vi "labview4.vi"() -> ()   [LabVIEW 2019]
uses:
  <vilib>/addons/eal4LabVIEW/ApiLib/Connection control/ealApiConnect_string.vi
  <vilib>/Utility/inputDevices.llb/joystickAcquire.vi
  <vilib>/Utility/inputDevices.llb/closeJoystick.vi
  <vilib>/addons/eal4LabVIEW/eal4LabVIEW.lvlib
panel:
  out "appended array":bool[](array[boolean])
  out "In Range? (1)":bool
  out "In Range? (2)":bool
  out "In Range? (3)":bool
  in  "condition 6":i32(ring) items=["AXIS_CONDITION_ACTIVE"=0, "AXIS_CONDITION_PARKING"=1, "AXIS_CONDITION_DEACTIVATED"=2, "AXIS_CONDITION_ACTIVE_DECOUPLED"=4, "AXIS_CONDITION_PARKING_DECOUPLED"=5, "AXIS_CONDITION_DEACTIVATED_DECOUPLED"=6, "AXIS_CONDITION_ACTIVE_PARAMETERIZATION"=8, "AXIS_CONDITION_PARKING_PARAMETERIZATION"=9, "AXIS_CONDITION_DEACTIVATED_PARAMETERIZATION"=10, "AXIS_CONDITION_ACTIVE_DECOUPLED_PARAMETERIZATION"=12, "AXIS_CONDITION_PARKING_DECOUPLED_PARAMETERIZATION"=13, "AXIS_CONDITION_DEACTIVATED_DECOUPLED_PARAMETERIZATION"=14]
  in  "slave index 6":i32
  in  "condition 5":i32(ring) items=["AXIS_CONDITION_ACTIVE"=0, "AXIS_CONDITION_PARKING"=1, "AXIS_CONDITION_DEACTIVATED"=2, "AXIS_CONDITION_ACTIVE_DECOUPLED"=4, "AXIS_CONDITION_PARKING_DECOUPLED"=5, "AXIS_CONDITION_DEACTIVATED_DECOUPLED"=6, "AXIS_CONDITION_ACTIVE_PARAMETERIZATION"=8, "AXIS_CONDITION_PARKING_PARAMETERIZATION"=9, "AXIS_CONDITION_DEACTIVATED_PARAMETERIZATION"=10, "AXIS_CONDITION_ACTIVE_DECOUPLED_PARAMETERIZATION"=12, "AXIS_CONDITION_PARKING_DECOUPLED_PARAMETERIZATION"=13, "AXIS_CONDITION_DEACTIVATED_DECOUPLED_PARAMETERIZATION"=14]
  in  "slave index 5":i32
  in  "condition 4":i32(ring) items=["AXIS_CONDITION_ACTIVE"=0, "AXIS_CONDITION_PARKING"=1, "AXIS_CONDITION_DEACTIVATED"=2, "AXIS_CONDITION_ACTIVE_DECOUPLED"=4, "AXIS_CONDITION_PARKING_DECOUPLED"=5, "AXIS_CONDITION_DEACTIVATED_DECOUPLED"=6, "AXIS_CONDITION_ACTIVE_PARAMETERIZATION"=8, "AXIS_CONDITION_PARKING_PARAMETERIZATION"=9, "AXIS_CONDITION_DEACTIVATED_PARAMETERIZATION"=10, "AXIS_CONDITION_ACTIVE_DECOUPLED_PARAMETERIZATION"=12, "AXIS_CONDITION_PARKING_DECOUPLED_PARAMETERIZATION"=13, "AXIS_CONDITION_DEACTIVATED_DECOUPLED_PARAMETERIZATION"=14]
  in  "slave index 4":i32
  out "RPM Motor 1":dbl
  out "RPM Motor 2":dbl
  out "RPM Motor 3":dbl
  in  "stop":bool
  out "return value":dbl[](array[numeric])
  out "Iteration counter":i32
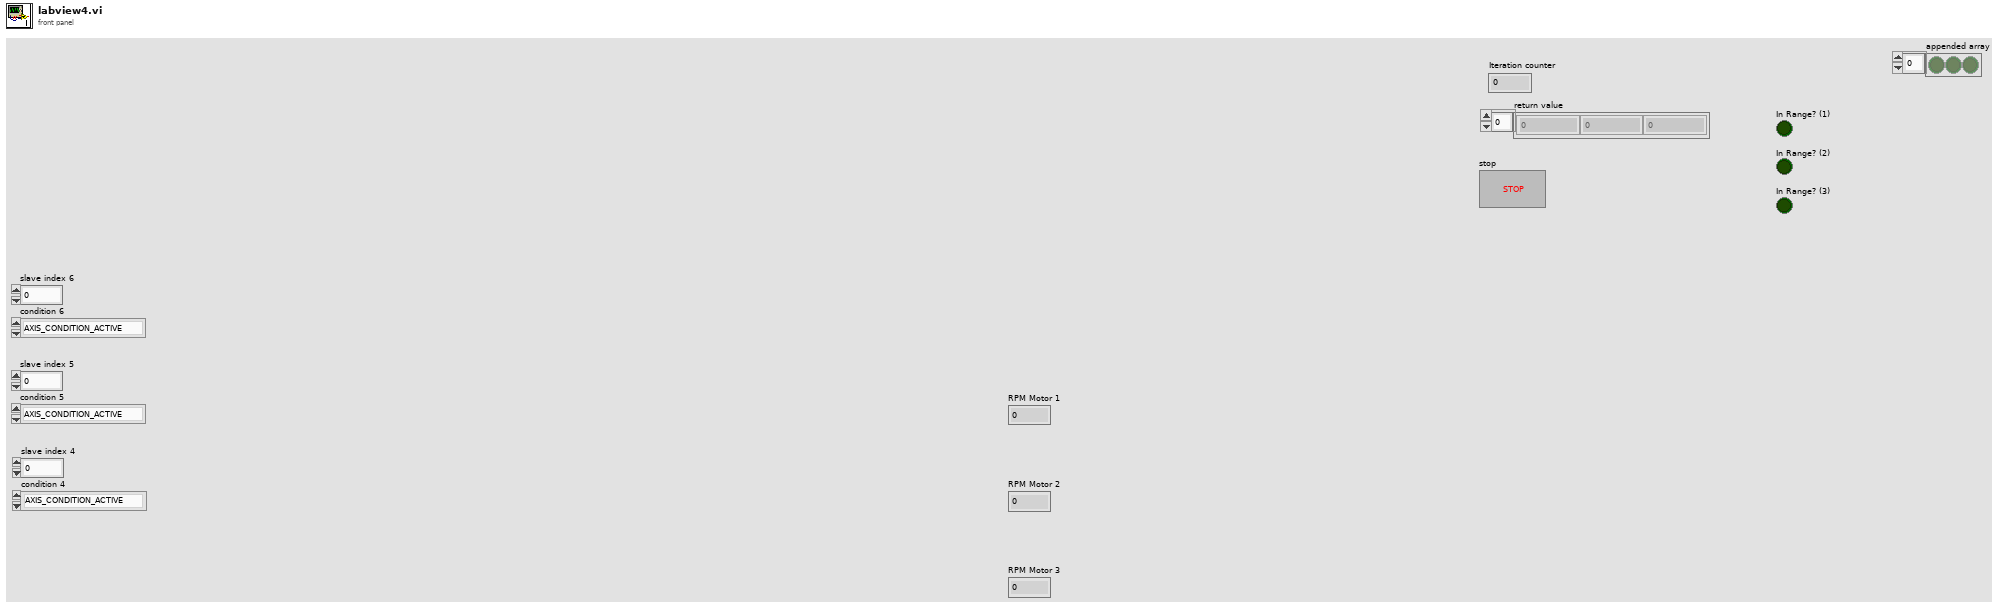
[diagram p1: front panel]
types:
  T1 = cluster{"Velocity":dbl, "Acceleration":dbl, "Deceleration":dbl, "Jerk":dbl}
  T2 = cluster{"X axis":i32, "Y axis":i32, "Z axis":i32, "X axis rotation":i32, "Y axis rotation":i32, "Z axis rotation":i32, "U axis":i32, "V axis":i32}
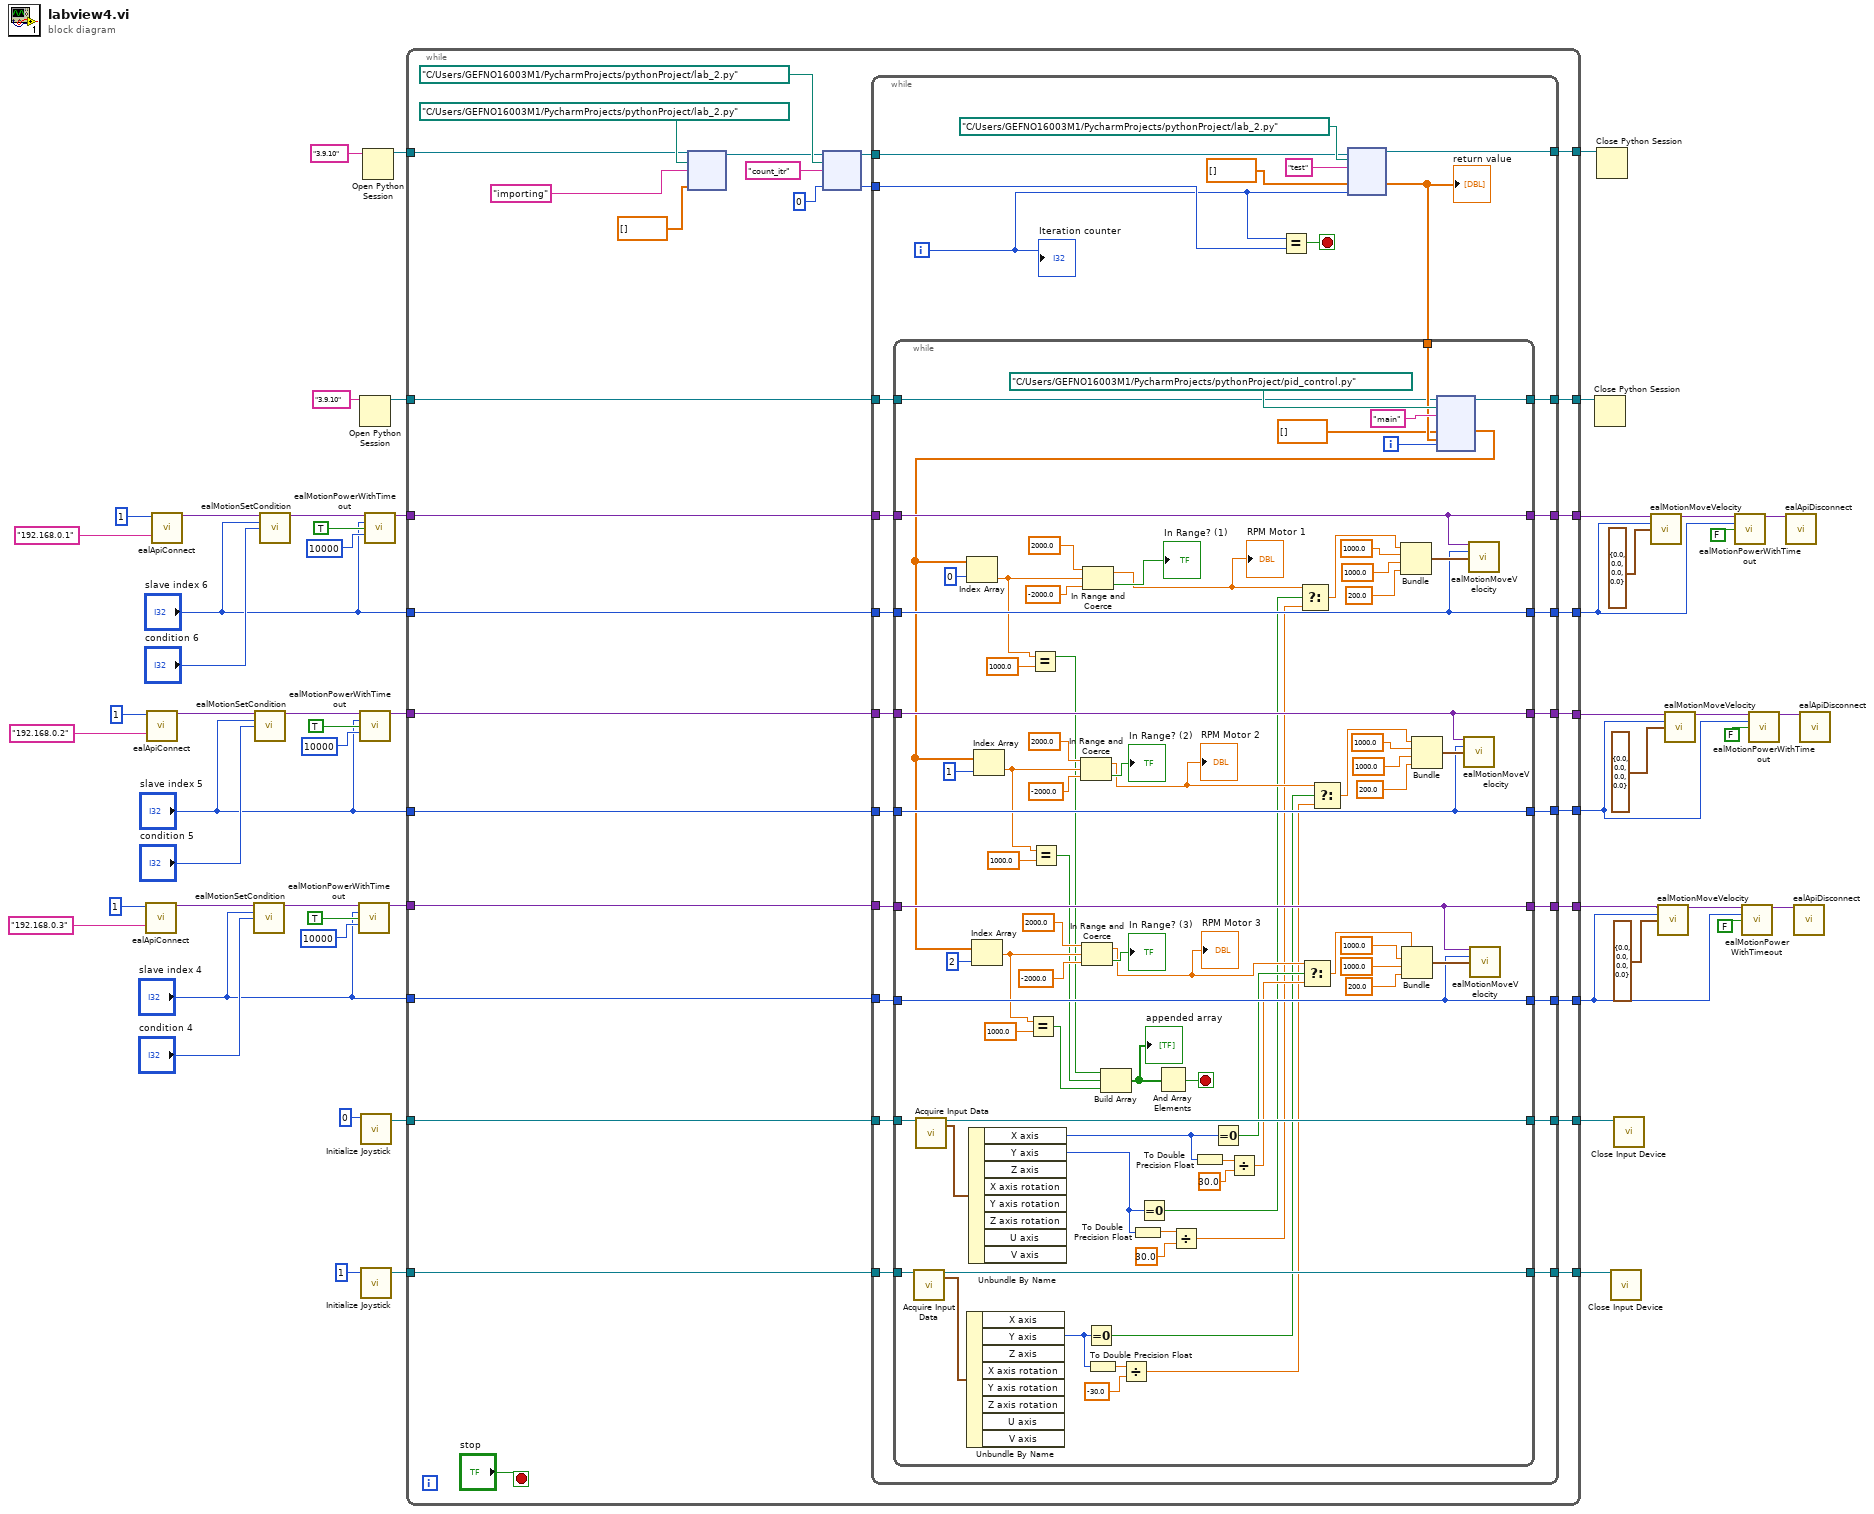
[diagram p0: block diagram]
diagram:
  n1 = call-poly <vilib>:"ealApiConnect.vi"("maximum no of axes"=1, "ip address"="192.168.0.3") -> ("connection out"=w43:variant)  [unwired: 12 in, 1 out]
  n2 = call-poly <vilib>:"ealApiConnect.vi"("maximum no of axes"=1, "ip address"="192.168.0.2") -> ("connection out"=w36:variant)  [unwired: 12 in, 1 out]
  n3 = call-poly <vilib>:"ealApiConnect.vi"("maximum no of axes"=1, "ip address"="192.168.0.1") -> ("connection out"=w29:variant)  [unwired: 12 in, 1 out]
  n4 = call <vilib>:"ealMotionSetCondition.vi"("connection in"=w43, "slave index"="slave index 4", "condition"="condition 4") -> ("connection out"=w42:variant)  [unwired: 11 in, 1 out]
  n5 = call <vilib>:"ealMotionSetCondition.vi"("connection in"=w36, "slave index"="slave index 5", "condition"="condition 5") -> ("connection out"=w35:variant)  [unwired: 11 in, 1 out]
  n6 = call <vilib>:"ealMotionSetCondition.vi"("connection in"=w29, "slave index"="slave index 6", "condition"="condition 6") -> ("connection out"=w28:variant)  [unwired: 11 in, 1 out]
  n7 = call <vilib>:"ealMotionPowerWithTimeout.vi"("connection in"=w42, "slave index"="slave index 4", "value"=TRUE, "timeout"=10000) -> ("connection out"=w22:variant)  [unwired: 10 in, 1 out]
  n8 = Open Python Session(python version="3.9.10" ("Python version")) -> (session out=w10:refnum<k35>)  [unwired: 2 in, 1 out]
  n9 = call <vilib>:"ealMotionPowerWithTimeout.vi"("connection in"=w35, "slave index"="slave index 5", "value"=TRUE, "timeout"=10000) -> ("connection out"=w23:variant)  [unwired: 10 in, 1 out]
  n10 = call <vilib>:"Initialize Joystick.vi"("device index"=0) -> ("device ID"=w4:refnum<k1>)  [unwired: 9 in, 1 out]
  n11 = call <vilib>:"Initialize Joystick.vi"("device index"=1) -> ("device ID"=w3:refnum<k1>)  [unwired: 9 in, 1 out]
  n12 = Open Python Session(python version="3.9.10" ("Python version")) -> (session out=w13:refnum<k35>)  [unwired: 2 in, 1 out]
  n13 = call <vilib>:"ealMotionPowerWithTimeout.vi"("connection in"=w28, "slave index"="slave index 6", "value"=TRUE, "timeout"=10000) -> ("connection out"=w24:variant)  [unwired: 10 in, 1 out]
  n14 = while {
    tunnel: w24 -> [w77]
    tunnel: w23 -> [w76]
    tunnel: w22 -> [w75]
    tunnel: [w74] -> w21
    tunnel: [w73] -> w20
    tunnel: "slave index 6" -> [w72]
    tunnel: "slave index 5" -> [w71]
    tunnel: [w70] -> w17
    tunnel: [w63] -> w16
    tunnel: "slave index 4" -> [w69]
    tunnel: w13 -> [w68]
    tunnel: [w67] -> w12
    tunnel: w10 -> [w66]
    tunnel: [w65] -> w9
    tunnel: [w64] -> w8
    tunnel: [w62] -> w7
    tunnel: w4 -> [w61]
    tunnel: w3 -> [w60]
    tunnel: [w59] -> w2
    tunnel: [w58] -> w1
    stop <- "stop" stop-if-true
    n15 = node(w68, path "C:/Users/GEFNO16003M1/PycharmProjects/pythonProject/lab_2.py" ("module path"), "importing" ("function name"), dbl[] []) -> (w82:refnum<k35>)  [unwired: 2 in, 3 out]
    n16 = node(w82, path "C:/Users/GEFNO16003M1/PycharmProjects/pythonProject/lab_2.py" ("module path"), "count_itr" ("function name"), 0) -> (w81:refnum<k35>, w79:i32)  [unwired: 1 in, 3 out]
    n17 = while {
      tunnel: [w108] -> w67
      tunnel: w81 -> [w111]
      tunnel: w79 -> [w109]
      tunnel: w77 -> [w106]
      tunnel: w76 -> [w95]
      tunnel: w75 -> [w105]
      tunnel: [w97] -> w74
      tunnel: [w98] -> w73
      tunnel: w72 -> [w96]
      tunnel: w71 -> [w94]
      tunnel: [w99] -> w70
      tunnel: w69 -> [w101]
      tunnel: w66 -> [w93]
      tunnel: [w103] -> w65
      tunnel: [w102] -> w64
      tunnel: [w100] -> w63
      tunnel: [w92] -> w62
      tunnel: w61 -> [w91]
      tunnel: w60 -> [w90]
      tunnel: [w89] -> w59
      tunnel: [w88] -> w58
      i -> [w104]
      stop <- w112 stop-if-true
      n18 = Equal?(x=w104, y=w109) -> (x = y?=w112:bool)
      n19 = node(w111, path "C:/Users/GEFNO16003M1/PycharmProjects/pythonProject/lab_2.py" ("module path"), "test" ("function name"), dbl[] [], w104) -> (w108:refnum<k35>, w107:dbl[])  [unwired: 2 in, 3 out]
      "return value" <- w107
      n20 = while {
        tunnel: w107 -> [w188]
        tunnel: w106 -> [w160]
        tunnel: w105 -> [w162]
        tunnel: [w162] -> w103
        tunnel: [w161] -> w102
        tunnel: w101 -> [w161]
        tunnel: [w158] -> w100
        tunnel: [w157] -> w99
        tunnel: [w159] -> w98
        tunnel: [w160] -> w97
        tunnel: w96 -> [w159]
        tunnel: w95 -> [w158]
        tunnel: w94 -> [w157]
        tunnel: w93 -> [w156]
        tunnel: [w155] -> w92
        tunnel: w91 -> [w141]
        tunnel: w90 -> [w140]
        tunnel: [w139] -> w89
        tunnel: [w138] -> w88
        i -> [w154]
        stop <- w152 stop-if-true
        n21 = call-poly <vilib>:"Acquire Input Data.vi"("device ID"=w140) -> ("device ID"=w138:refnum<k1>, "axis info"=w136:T2)  [unwired: 14 in, 3 out]
        n22 = call-poly <vilib>:"Acquire Input Data.vi"("device ID"=w141) -> ("device ID"=w139:refnum<k1>, "axis info"=w137:T2)  [unwired: 14 in, 3 out]
        n23 = Unbundle By Name(w136) -> ("Y axis"=w125:i32)  [unwired: 7 out]
        n24 = Unbundle By Name(w137) -> ("X axis"=w133:i32, "Y axis"=w132:i32)  [unwired: 6 out]
        n25 = Equal To 0?(x=w125) -> (x = 0?=w120:bool)
        n26 = To Double Precision Float(number=w125) -> (double precision float=w126:dbl)
        n27 = Divide(x=w126, y=-30.0) -> (x/y=w119:dbl)
        n28 = To Double Precision Float(number=w132) -> (double precision float=w124:dbl)
        n29 = Equal To 0?(x=w132) -> (x = 0?=w116:bool)
        n30 = Divide(x=w124, y=30.0) -> (x/y=w115:dbl)
        n31 = To Double Precision Float(number=w133) -> (double precision float=w130:dbl)
        n32 = Equal To 0?(x=w133) -> (x = 0?=w131:bool)
        n33 = Divide(x=w130, y=30.0) -> (x/y=w128:dbl)
        n34 = node(w156, path "C:/Users/GEFNO16003M1/PycharmProjects/pythonProject/pid_control.py" ("module path"), "main" ("function name"), dbl[] [], w188, w154) -> (w155:refnum<k35>, w153:dbl[])  [unwired: 3 in, 3 out]
        n35 = Index Array(array=w153, index=0) -> (element=w148:dbl)
        n36 = Index Array(array=w153, index=2) -> (element=w146:dbl)
        n37 = Index Array(array=w153, index=1) -> (element=w147:dbl)
        n38 = Equal?(x=w146, y=1000.0) -> (x = y?=w143:bool)
        n39 = Equal?(x=w148, y=1000.0) -> (x = y?=w145:bool)
        n40 = Equal?(x=w147, y=1000.0) -> (x = y?=w144:bool)
        n41 = In Range and Coerce(upper limit=2000.0, x=w147, lower limit=-2000.0) -> (coerced(x)=w121:dbl, In Range?=→"In Range? (2)":bool)
        "RPM Motor 2" <- w121
        n42 = In Range and Coerce(upper limit=2000.0, x=w146, lower limit=-2000.0) -> (coerced(x)=w134:dbl, In Range?=→"In Range? (3)":bool)
        "RPM Motor 3" <- w134
        n43 = In Range and Coerce(upper limit=2000.0, x=w148, lower limit=-2000.0) -> (coerced(x)=w117:dbl, In Range?=→"In Range? (1)":bool)
        "RPM Motor 1" <- w117
        n44 = Build Array(w145, w144, w143) -> (w142:bool[])
        "appended array" <- w142
        n45 = And Array Elements(Boolean array=w142) -> (logical AND=w152:bool)
        n46 = Select(t=w117, s=w116, f=w115) -> (s? t:f=w118:dbl)
        n47 = Select(t=w134, s=w131, f=w128) -> (s? t:f=w135:dbl)
        n48 = Select(t=w121, s=w120, f=w119) -> (s? t:f=w122:dbl)
        n49 = Bundle("upper limit"=w118, 1000.0, 1000.0, 200.0) -> (w172:cluster{"upper limit":dbl, dbl, dbl, dbl})  [unwired: 1 in]
        n50 = Bundle("upper limit"=w135, 1000.0, 1000.0, 200.0) -> (w182:cluster{"upper limit":dbl, dbl, dbl, dbl})  [unwired: 1 in]
        n51 = Bundle("upper limit"=w122, 1000.0, 1000.0, 200.0) -> (w177:cluster{"upper limit":dbl, dbl, dbl, dbl})  [unwired: 1 in]
        n52 = call <vilib>:"ealMotionMoveVelocity.vi"("connection in"=w158, "slave index"=w157, "parameters set"=w177) -> ()  [unwired: 11 in, 2 out]
        n53 = call <vilib>:"ealMotionMoveVelocity.vi"("connection in"=w160, "slave index"=w159, "parameters set"=w172) -> ()  [unwired: 11 in, 2 out]
        n54 = call <vilib>:"ealMotionMoveVelocity.vi"("connection in"=w162, "slave index"=w161, "parameters set"=w182) -> ()  [unwired: 11 in, 2 out]
      }
      "Iteration counter" <- w104
    }
  }
  n55 = Close Python Session(session in=w7) -> ()  [unwired: 1 in, 1 out]
  n56 = Close Python Session(session in=w12) -> ()  [unwired: 1 in, 1 out]
  n57 = call-poly <vilib>:"Close Input Device.vi"("device ID"=w1) -> ()  [unwired: 9 in, 1 out]
  n58 = call-poly <vilib>:"Close Input Device.vi"("device ID"=w2) -> ()  [unwired: 9 in, 1 out]
  n59 = call <vilib>:"ealMotionMoveVelocity.vi"("connection in"=w21, "slave index"=w20, "parameters set"=T1 {"Velocity"=0.0, "Acceleration"=0.0, "Deceleration"=0.0, "Jerk"=0.0}) -> ("connection out"=w48:variant)  [unwired: 11 in, 1 out]
  n60 = call <vilib>:"ealMotionMoveVelocity.vi"("connection in"=w9, "slave index"=w8, "parameters set"=T1 {"Velocity"=0.0, "Acceleration"=0.0, "Deceleration"=0.0, "Jerk"=0.0}) -> ("connection out"=w56:variant)  [unwired: 11 in, 1 out]
  n61 = call <vilib>:"ealMotionMoveVelocity.vi"("connection in"=w16, "slave index"=w17, "parameters set"=T1 {"Velocity"=0.0, "Acceleration"=0.0, "Deceleration"=0.0, "Jerk"=0.0}) -> ("connection out"=w52:variant)  [unwired: 11 in, 1 out]
  n62 = call <vilib>:"ealMotionPowerWithTimeout.vi"("connection in"=w48, "slave index"=w20, "value"=FALSE) -> ("connection out"=w49:variant)  [unwired: 11 in, 1 out]
  n63 = call <vilib>:"ealMotionPowerWithTimeout.vi"("connection in"=w56, "slave index"=w8, "value"=FALSE) -> ("connection out"=w57:variant)  [unwired: 11 in, 1 out]
  n64 = call <vilib>:"ealMotionPowerWithTimeout.vi"("connection in"=w52, "slave index"=w17, "value"=FALSE) -> ("connection out"=w53:variant)  [unwired: 11 in, 1 out]
  n65 = call <vilib>:"ealApiDisconnect.vi"("connection in"=w49) -> ()  [unwired: 14 in, 1 out]
  n66 = call <vilib>:"ealApiDisconnect.vi"("connection in"=w57) -> ()  [unwired: 14 in, 1 out]
  n67 = call <vilib>:"ealApiDisconnect.vi"("connection in"=w53) -> ()  [unwired: 14 in, 1 out]
